vi "PositionToReceivePass2ndStrikerDoublePass.vi"(6 "TimeElapsed?":bool=TRUE, 7 "Boolean":bool=TRUE, 8 "error in (no error)":errorcluster, 9 "Game":refnum<class "Game.lvclass">, 10 "Robot":refnum<class "Robot.lvclass">, 11 "PositionToReceivePassSkill in":refnum<class "PositionToReceivePassSkill.lvclass">) -> (0 "error out":errorcluster, 2 "2ndStrikerPositionDoublePass":dbl[](array[numeric]), 3 "PositionToReceivePassSkill out":refnum<class "PositionToReceivePassSkill.lvclass">)   [LabVIEW 2020, in "PositionToReceivePassSkill.lvclass"]
uses:
  PositionToReceivePassSkill.lvclass
  Game_class/Game.lvclass
  Robot_class/Robot.lvclass
  Game_class/Game.lvclass/Game.ctl
  Parameters_class/Parameters.lvclass/Parameters.ctl
  Object_class/Object.lvclass/Object.ctl
  Game_class/Read Utilities.lvclass.vi
  Game_class/Read Parameters.lvclass.vi
  Game_class/Read FieldRef.vi
  Game_class/Read BallRef.vi
  Object_class/Read x.vi
  Object_class/Read y.vi
  Parameters_class/Read AttakingOurselves.vi
  Ball_class/Ball.lvclass
  C:/Users/pipew/OneDrive/Documentos/GitHub/SSL_AI/Object_class/Object.lvclass
  Utilities_class/Utilities.lvclass
  Parameters_class/Parameters.lvclass
  Field_class/Field.lvclass
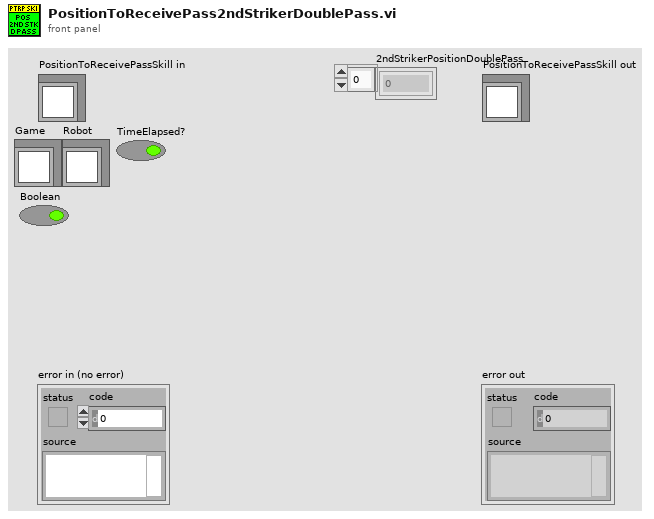
[diagram p1: front panel]
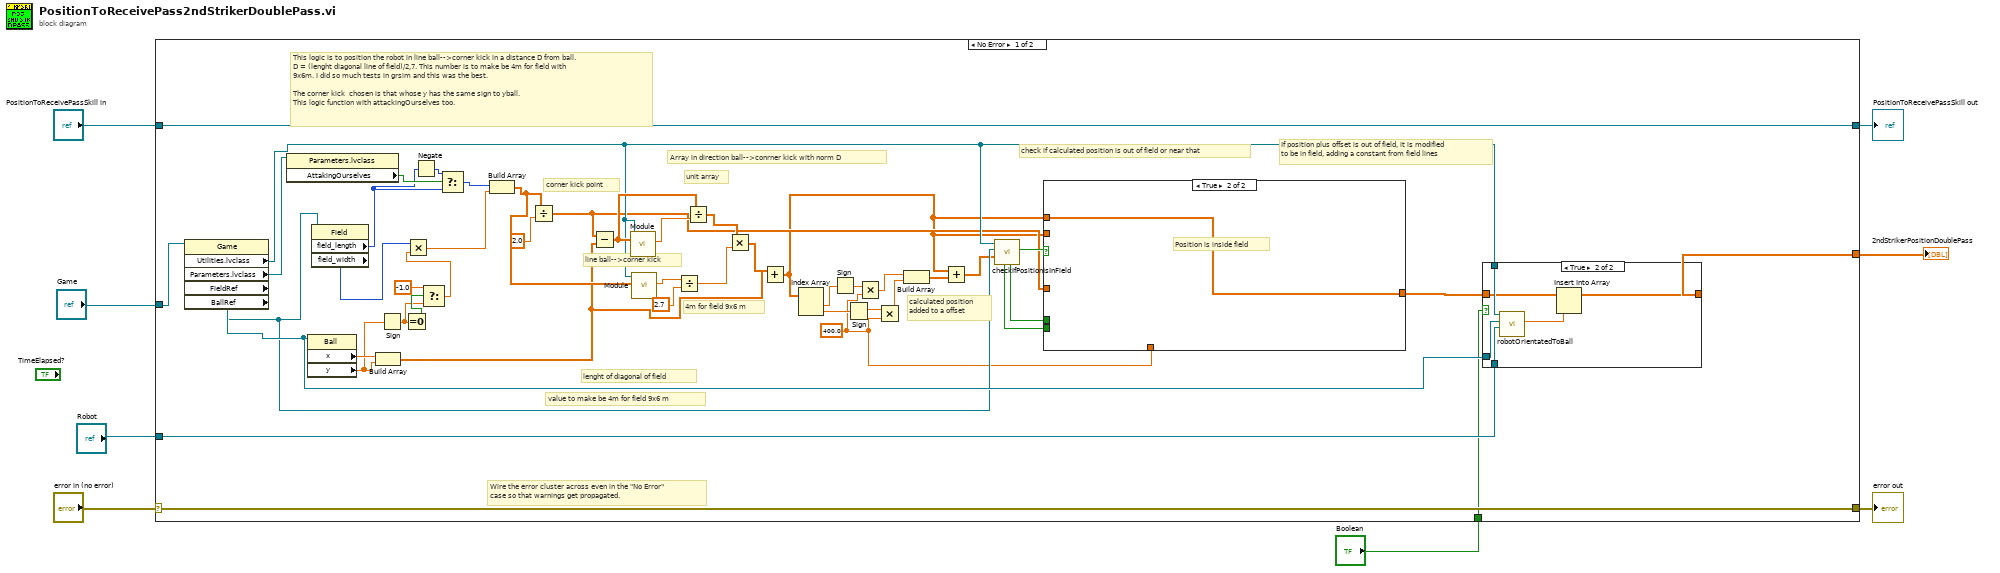
[diagram p0: block diagram]
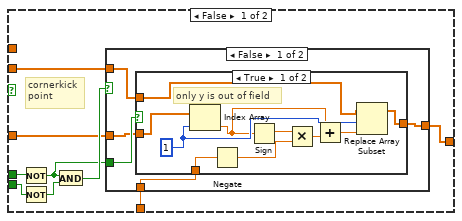
[diagram p3: hidden frame]
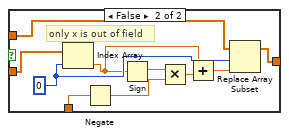
[diagram p4: hidden frame]
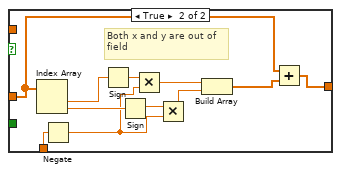
[diagram p5: hidden frame]
diagram:
  n1 = case shown="No Error" "error in (no error)" {
    selector: "error in (no error)" -> [w54 w110]
    tunnel: [w54 w110] -> w7
    tunnel: [w55 w109] -> w5
    tunnel: "PositionToReceivePassSkill in" -> [w55 w109]
    tunnel: "Game" -> [w23 _]
    tunnel: "Robot" -> [w34 _]
    tunnel: [w32 _] -> w2
    tunnel: "Boolean" -> [w9 _]
    frame No Error {
      w16 = 400.0 ("y")
      # "If position plus offset is out of field, it is modified\nto be in field, adding a constant from field lines"
      # "calculated position\nadded to a offset"
      # "check if calculated position is out of field or near that"
      # "Array in direction ball-->conrner kick with norm D"
      # "This logic is to position the robot in line ball-->corner kick in a distance D from ball.\nD = (lenght diagonal line of field)/2,7. This number is to make be 4m for field with\n9x6m. I did so much tests in grsim and this was the best.\n\nThe corner kick  chosen is that whose y has the same sign to yball.\nThis logic function with attackingOurselves too."
      # "value to make be 4m for field 9x6 m"
      # "4m for field 9x6 m"
      # "lenght of diagonal of field"
      # "unit array"
      # "line ball-->corner kick"
      # "corner kick point"
      # "Wire the error cluster across even in the \"No Error\"\ncase so that warnings get propagated."
      n2 = property class="Game"(reference=w23) -> ("Utilities.lvclass"=w24:refnum<class "Utilities.lvclass">, "Parameters.lvclass"=w50:refnum<class "Parameters.lvclass">, "FieldRef"=w22:refnum<class "Field.lvclass">, "BallRef"=w33:refnum<class "Ball.lvclass">)  [unwired: 1 in, 2 out]
      n3 = property class="Parameters.lvclass"(reference=w50) -> ("AttakingOurselves"=w49:bool)  [unwired: 1 in, 2 out]
      n4 = property class="Ball"(reference=w33) -> ("x"=w53:dbl, "y"=w51:dbl)  [unwired: 1 in, 2 out]
      n5 = property class="Field"(reference=w22) -> ("field_length"=w47:i32, "field_width"=w52:i32)  [unwired: 1 in, 2 out]
      n6 = Build Array(w53, w51) -> (w35:dbl[])
      n7 = Sign(1:w51) -> (0:w12:dbl)
      n8 = Equal To 0?(x=w12) -> (x = 0?=w13:bool)
      n9 = Negate(x=w47) -> (-x=w48:i32)
      n10 = Select(t=-1.0, s=w13, f=w12) -> (s? t:f=w10:dbl)
      n11 = Multiply(x=w52, y=w10) -> (x*y=w45:dbl)
      n12 = Select(t=w48, s=w49, f=w47) -> (s? t:f=w46:i32)
      n13 = Build Array(w46, w45) -> (w40:dbl[])
      n14 = Divide(x=w40, y=2.0) -> (x/y=w17:dbl[])
      n15 = Subtract(x=w17, y=w35) -> (x-y=w43:dbl[])
      n16 = call-dynamic "Module.vi"("2D vector"=w43, "Utilities in"=w24) -> ("Modulo"=w42:dbl)  [unwired: 7 in, 2 out]
      n17 = call-dynamic "Module.vi"("2D vector"=w40, "Utilities in"=w24) -> ("Modulo"=w39:dbl)  [unwired: 7 in, 2 out]
      n18 = Divide(x=w39, y=2.7) -> (x/y=w37:dbl)
      n19 = Divide(x=w43, y=w42) -> (x/y=w41:dbl[])
      n20 = Multiply(x=w41, y=w37) -> (x*y=w36:dbl[])
      n21 = Add(x=w36, y=w35) -> (x+y=w15:dbl[])
      n22 = Index Array(array=w15) -> (element #1=w31:dbl, element #2=w28:dbl)  [unwired: 2 in]
      n23 = Sign(1:w31) -> (0:w30:dbl)
      n24 = Sign(1:w28) -> (0:w29:dbl)
      n25 = Multiply(x=w30, y=w16) -> (x*y=w27:dbl)
      n26 = Multiply(x=w29, y=w16) -> (x*y=w26:dbl)
      n27 = Build Array(w27, w26) -> (w25:dbl[])
      n28 = Add(x=w15, y=w25) -> (x+y=w14:dbl[])
      n29 = call "checkIfPositionIsInField.vi"("Position"=w14, "FieldRef"=w22, "Utilities in"=w24) -> ("Position Is In Field?"=w21:bool, "y Is in Field?"=w19:bool, "x Is in Field?"=w18:bool)  [unwired: 4 in, 2 out]
      n30 = case shown="True" w21 {
        tunnel: w15 -> [_ w108]
        tunnel: [w65 w108] -> w20
        tunnel: w19 -> [w70 _]
        tunnel: w18 -> [w69 _]
        tunnel: w17 -> [w67 _]
        tunnel: w16 -> [w66 _]
        tunnel: w15 -> [w63 _]
        frame False {
          # "cornerkick\npoint"
          n31 = Not(x=w70) -> (.not. x?=w64:bool)
          n32 = Not(x=w69) -> (.not. x?=w68:bool)
          n33 = And(x=w64, y=w68) -> (x .and. y?=w71:bool)
          n34 = case shown="False" w71 {
            tunnel: w67 -> [w72 w98]
            tunnel: w66 -> [w75 w100]
            tunnel: [w74 w97] -> w65
            tunnel: w64 -> [w76 _]
            tunnel: w63 -> [w73 _]
            frame False {
              n35 = case shown="True" w76 {
                tunnel: w73 -> [w77 w88]
                tunnel: w75 -> [w84 w94]
                tunnel: [w82 w92] -> w74
                tunnel: w72 -> [w78 w87]
                frame True {
                  w83 = 1
                  # "only y is out of field"
                  n36 = Index Array(array=w78, index=w83) -> (element=w79:dbl)
                  n37 = Negate(x=w84) -> (-x=w85:dbl)
                  n38 = Sign(1:w79) -> (0:w86:dbl)
                  n39 = Multiply(x=w86, y=w85) -> (x*y=w81:dbl)
                  n40 = Add(x=w79, y=w81) -> (x+y=w80:dbl)
                  n41 = Replace Array Subset(array=w77, new element=w80, index=w83) -> (w82:dbl[])
                }
                frame False {
                  w93 = 0
                  # "only x is out of field"
                  n42 = Index Array(array=w87, index=w93) -> (element=w89:dbl)
                  n43 = Negate(x=w94) -> (-x=w95:dbl)
                  n44 = Sign(1:w89) -> (0:w96:dbl)
                  n45 = Multiply(x=w96, y=w95) -> (x*y=w91:dbl)
                  n46 = Add(x=w89, y=w91) -> (x+y=w90:dbl)
                  n47 = Replace Array Subset(array=w88, new element=w90, index=w93) -> (w92:dbl[])
                }
              }
            }
            frame True {
              # "Both x and y are out of\nfield"
              n48 = Index Array(array=w98) -> (element #1=w107:dbl, element #2=w104:dbl)  [unwired: 2 in]
              n49 = Negate(x=w100) -> (-x=w101:dbl)
              n50 = Sign(1:w107) -> (0:w106:dbl)
              n51 = Sign(1:w104) -> (0:w105:dbl)
              n52 = Multiply(x=w106, y=w101) -> (x*y=w103:dbl)
              n53 = Multiply(x=w105, y=w101) -> (x*y=w102:dbl)
              n54 = Build Array(w103, w102) -> (w99:dbl[])
              n55 = Add(x=w98, y=w99) -> (x+y=w97:dbl[])
            }
          }
        }
        frame True {
          # "Position is inside field"
        }
      }
      n56 = case shown="True" w9 {
        tunnel: w34 -> [_ w61]
        tunnel: w33 -> [_ w60]
        tunnel: [w56 w59] -> w32
        tunnel: w24 -> [_ w58]
        tunnel: w20 -> [w56 w57]
        frame False {
        }
        frame True {
          n57 = call "robotOrientatedToBall.vi"("Robot"=w61, "BallRef"=w60, "Utilities in"=w58) -> ("Orientation"=w62:dbl)  [unwired: 6 in, 2 out]
          n58 = Insert Into Array(array=w57, new element=w62) -> (w59:dbl[])  [unwired: 1 in]
        }
      }
    }
    frame Error {
    }
  }
  "error out" <- w7
  "PositionToReceivePassSkill out" <- w5
  "2ndStrikerPositionDoublePass" <- w2
